vi "SLSCTest Parsing Capabilities Files.vi"() -> (3 "Test passed?":bool)   [LabVIEW 2015, in "SLSC EDS Testing.lvlib"]
uses:
  SLSC EDS Testing.lvlib
  SLSC EDS API/JSON parsing/EDSjsonStructure.ctl
  SLSC EDS API/JSON parsing/enum.ctl
  SLSC EDS API/JSON parsing/property.ctl
  SLSC EDS API/JSON parsing/command.ctl
  SLSC EDS API/JSON parsing/scale.ctl
  SLSC EDS API/JSON parsing/physicalChannel.ctl
  SLSC EDS API/JSON parsing/register.ctl
panel:
  out "appended array":path[](array[path])
  out "Array 2":errorcluster[](array[cluster])
  out "Array":T1[](array[typedef])
  # "not working\nregisterMap->registers->initialValue"
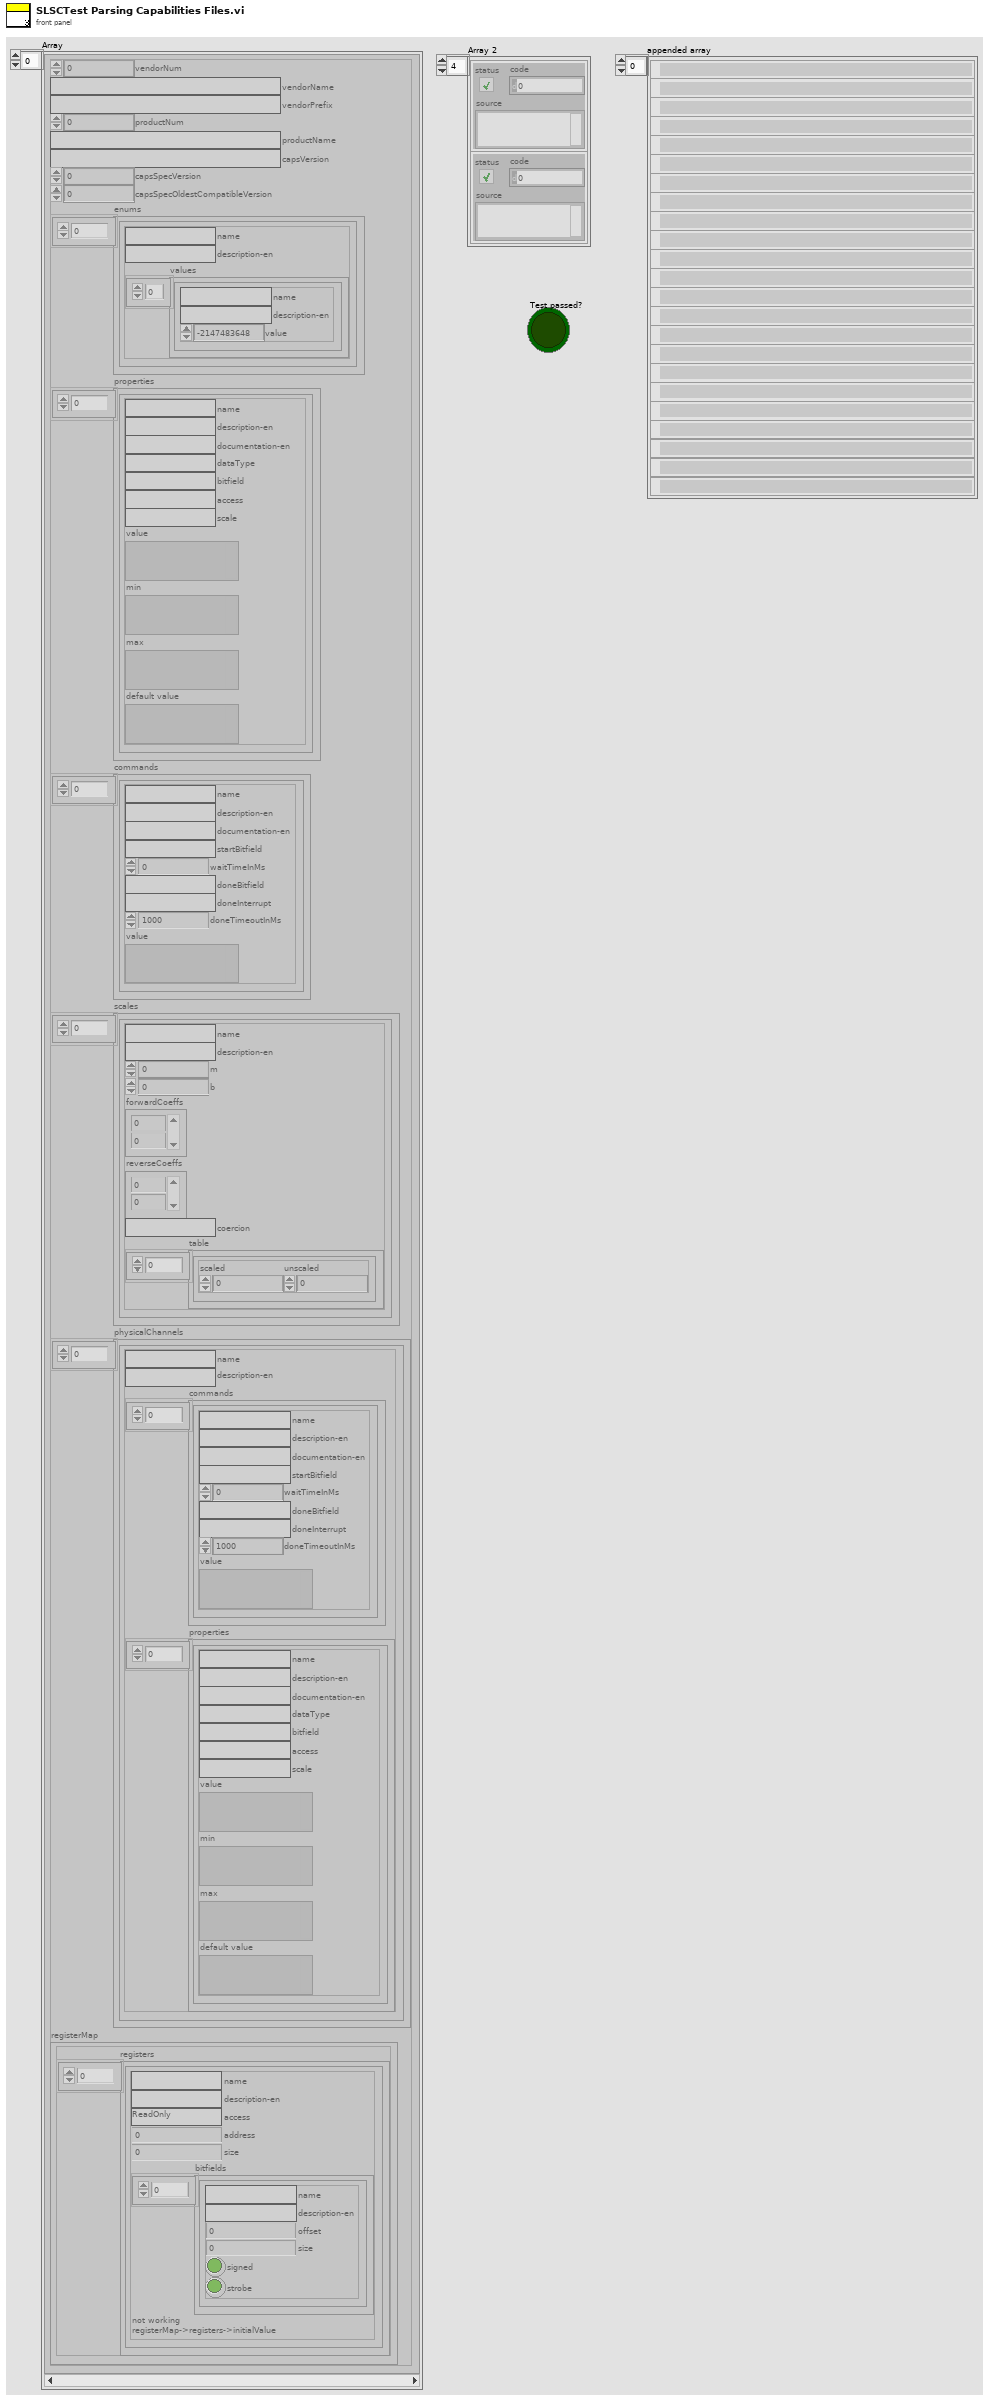
[diagram p1: front panel]
types:
  T1 = typedef "EDSjsonStructure.ctl" = cluster{"vendorNum":u32, "vendorName":string, "vendorPrefix":string, "productNum":u32, "productName":string, "capsVersion":string, "capsSpecVersion":u32, "capsSpecOldestCompatibleVersion":u32, "enums":T2[], "properties":T3[], "commands":T4[], "scales":T5[], "physicalChannels":T6[], "registerMap":cluster{"registers":T7[]}}
  T2 = typedef "enum.ctl" = cluster{"name":string, "description-en":string, "values":cluster{"name":string, "description-en":string, "value":i32}[]}
  T3 = typedef "property.ctl" = cluster{"name":string, "description-en":string, "documentation-en":string, "dataType":string, "bitfield":string, "access":string, "scale":string, "value":variant, "min":variant, "max":variant, "default value":variant}
  T4 = typedef "command.ctl" = cluster{"name":string, "description-en":string, "documentation-en":string, "startBitfield":string, "waitTimeInMs":i32, "doneBitfield":string, "doneInterrupt":string, "doneTimeoutInMs":i32, "value":variant}
  T5 = typedef "scale.ctl" = cluster{"name":string, "description-en":string, "m":dbl, "b":dbl, "forwardCoeffs":dbl[], "reverseCoeffs":dbl[], "coercion":string, "table":cluster{"scaled":dbl, "unscaled":dbl}[]}
  T6 = typedef "physicalChannel.ctl" = cluster{"name":string, "description-en":string, "commands":T4[], "properties":T3[]}
  T7 = typedef "register.ctl" = cluster{"name":string, "description-en":string, "access":string, "address":u32, "size":u32, "bitfields":cluster{"name":string, "description-en":string, "offset":u32, "size":u32, "signed":bool, "strobe":bool}[]}
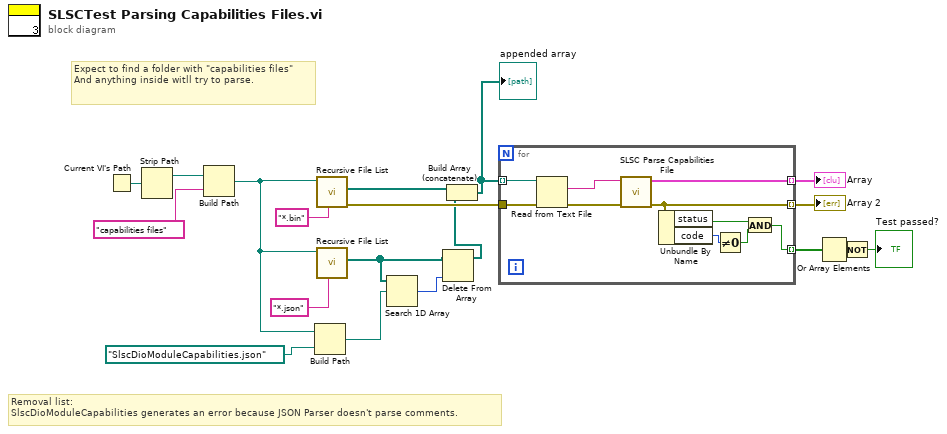
[diagram p0: block diagram]
diagram:
  # "Expect to find a folder with \"capabilities files\" \nAnd anything inside witll try to parse."
  # "Removal list:\nSlscDioModuleCapabilities generates an error because JSON Parser doesn't parse comments."
  n1 = Current VI's Path() -> (path=w19:path)
  n2 = Strip Path(path=w19) -> (stripped path=w5:path)  [unwired: 1 out]
  n3 = Build Path(base path=w5, name or relative path="capabilities files") -> (appended path=w2:path)
  n4 = Build Path(base path=w2, name or relative path=path "SlscDioModuleCapabilities.json" ("element")) -> (appended path=w1:path)
  n5 = call <vilib>:"Recursive File List.vi"("pattern"="*.bin", "Folder Path"=w2) -> ("error out"=w15:errorcluster, "All Files in Dir"=w17:path[])  [unwired: 5 in, 3 out]
  n6 = call <vilib>:"Recursive File List.vi"("pattern"="*.json", "Folder Path"=w2) -> ("All Files in Dir"=w9:path[])  [unwired: 5 in, 4 out]
  n7 = Search 1D Array(1D array=w9, element=w1) -> (index of element=w11:i32)  [unwired: 1 in]
  n8 = Delete From Array(array=w9, index=w11) -> (array with subset deleted=w6:path[])  [unwired: 1 in, 1 out]
  n9 = Build Array (concatenate)(w17, w6) -> (w13:path[])
  "appended array" <- w13
  n10 = for {
    tunnel: w13 -> [w29] mode=indexing
    tunnel: [w27] -> w16 mode=indexing
    tunnel: w15 -> [w26]
    tunnel: [w24] -> w14 mode=indexing
    tunnel: [w20] -> w10 mode=indexing
    n11 = Read from Text File(file (use dialog)=w29, error in=w26) -> (text=w28:string, error out=w25:errorcluster)  [unwired: 2 in, 2 out]
    n12 = call "SLSC Parse Capabilities File.vi"("error in"=w25, "module capabilities JSON string"=w28) -> ("error out"=w24:errorcluster, "SLSC EDS module"=w27:T1)  [unwired: 8 in]
    n13 = Unbundle By Name(w24) -> ("status"=w23:bool, "code"=w22:i32)
    n14 = Not Equal To 0?(x=w22) -> (x != 0?=w21:bool)
    n15 = And(x=w23, y=w21) -> (x .and. y?=w20:bool)
  }
  "Array" <- w16
  "Array 2" <- w14
  n16 = Or Array Elements(Boolean array=w10) -> (logical OR=w8:bool)
  n17 = Not(x=w8) -> (.not. x?=→"Test passed?":bool)
